vi "测试-已失败-调用python进行模型预测.vi"() -> ()   [LabVIEW 2018]
panel:
  out "output":T1(plugin-control)
  out "test":T1(plugin-control)
  out "图片路径名":path
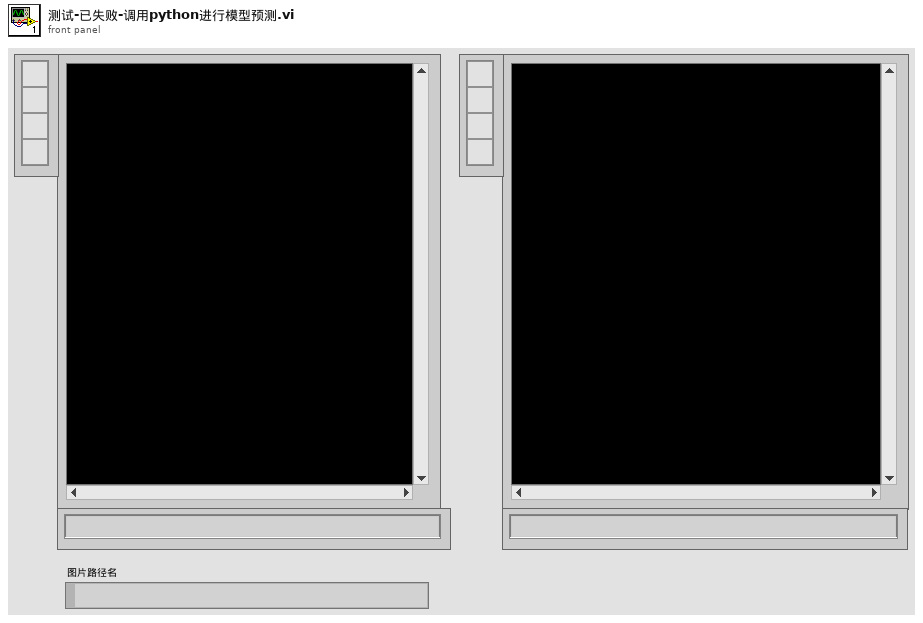
[diagram p1: front panel]
types:
  T1 = typedef "IMAQ Image.ctl" = refnum<image>
  T2 = typedef "Image Type" = u32
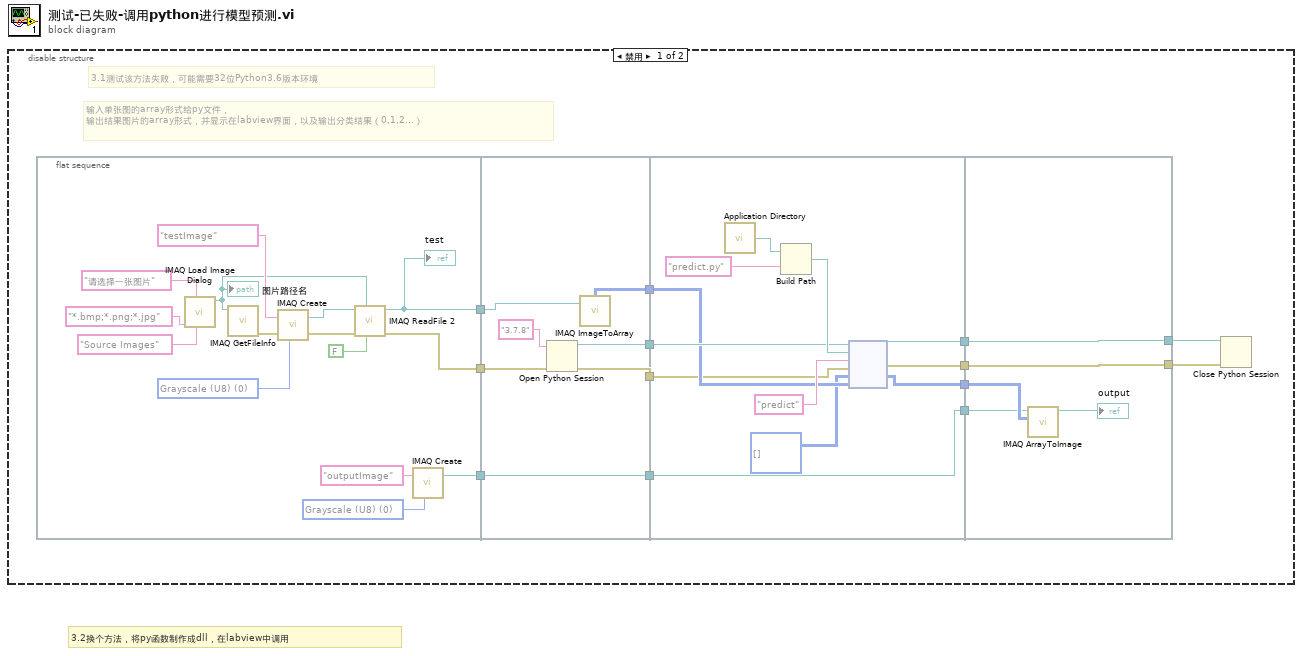
[diagram p0: block diagram]
diagram:
  # "3.2换个方法，将py函数制作成dll，在labview中调用"
  n1 = disable-structure shown="禁用" {
    frame Disabled {
      # "3.1测试该方法失败，可能需要32位Python3.6版本环境"
      # "输入单张图的array形式给py文件，\n输出结果图片的array形式，并显示在labview界面，以及输出分类结果（0,1,2...）"
      n2 = flat-sequence {
        tunnel: [w18] -> w13
        tunnel: [w17] -> w12
        tunnel: [w14] -> w11
        tunnel: w13 -> [w34]
        tunnel: [w33] -> w10
        tunnel: [w32] -> w9
        tunnel: [w31] -> w8
        tunnel: w12 -> [w30]
        tunnel: [w29] -> w7
        tunnel: w11 -> [w29]
        tunnel: w10 -> [w44]
        tunnel: w9 -> [w42]
        tunnel: [w41] -> w6
        tunnel: [w40] -> w5
        tunnel: w8 -> [w39]
        tunnel: [w38] -> w4
        tunnel: [w36] -> w3
        tunnel: w7 -> [w36]
        tunnel: w6 -> [w52]
        tunnel: w5 -> [w51]
        tunnel: [w52] -> w2
        tunnel: [w51] -> w1
        tunnel: w4 -> [w50]
        tunnel: w3 -> [w48]
        frame #0 {
          w16 = T2 0 items=["Grayscale (U8)", "Grayscale (I16)", "Grayscale (SGL)", "Complex (CSG)", "RGB (U32)", "HSL (U32)", "RGB (U64)", "Grayscale (U16)"] ("Image Type")
          w20 = T2 0 items=["Grayscale (U8)", "Grayscale (I16)", "Grayscale (SGL)", "Complex (CSG)", "RGB (U32)", "HSL (U32)", "RGB (U64)", "Grayscale (U16)"] ("Image Type")
          n3 = call "IMAQ Load Image Dialog"("Pattern Label"="Source Images", "Prompt"="请选择一张图片" ("prompt"), "Pattern"="*.bmp;*.png;*.jpg") -> ("Path"=w19:path)  [unwired: 6 in, 2 out]
          "图片路径名" <- w19
          n4 = call "IMAQ GetFileInfo"("File Path"=w19) -> ("error out"=w23:errorcluster)  [unwired: 4 in, 6 out]
          n5 = call "IMAQ Create"("Image Name"="testImage", "Image Type"=w20, "error in (no error)"=w23) -> ("New Image"=w24:T1, "error out"=w25:errorcluster)  [unwired: 2 in]
          n6 = call "IMAQ ReadFile 2"("Use File Path Image Type"=FALSE, "File Path"=w19, "error in (no error)"=w25, "Image"=w24) -> ("error out"=w17:errorcluster, "Image Out"=w18:T1)  [unwired: 3 in, 3 out]
          "test" <- w18
          n7 = call "IMAQ Create"("Image Name"="outputImage", "Image Type"=w16) -> ("New Image"=w14:T1)  [unwired: 3 in, 1 out]
        }
        frame #1 {
          n8 = Open Python Session(python version="3.7.8" ("Python版本"), 3:w30) -> (session out=w33:refnum<k35>, error out=w31:errorcluster)  [unwired: 1 in]
          n9 = call "IMAQ ImageToArray"("Image"=w34) -> ("Image Pixels (U8)"=w32:u8[][])  [unwired: 3 in, 4 out]
        }
        frame #2 {
          n10 = call <vilib>:"Application Directory.vi"() -> ("Application Directory"=w47:path)
          n11 = Build Path(base path=w47, name or relative path="predict.py" ("名称或相对路径")) -> (appended path=w45:path)
          n12 = node(w44, w45, "predict" ("函数名称"), w39, i32[][] [], w42) -> (w41:refnum<k35>, w40:errorcluster, w38:i32[][])  [unwired: 1 in, 2 out]
        }
        frame #3 {
          n13 = call "IMAQ ArrayToImage"("Image Pixels (U8)"=w50, "Image"=w48) -> ("Image Out"=→"output":T1)  [unwired: 8 in, 1 out]
        }
      }
      n14 = Close Python Session(session in=w2, error in=w1) -> ()  [unwired: 1 out]
    }
    frame Enabled {
    }
  }
